vi "BuildHelpPath.vi"(1 "Help File Name":string="lvhelp.chm") -> (0 "Help File Path":path)   [LabVIEW 2018]
doc: "This VI appends the passed in file name to the help directory and returns the full path. Input defaults to LabVIEW's main help file when not supplied."
panel:
  # "This VI appends the passed in file name to the help directory and returns\nthe full path. Input defaults to LabVIEW's main help file when not supplied."
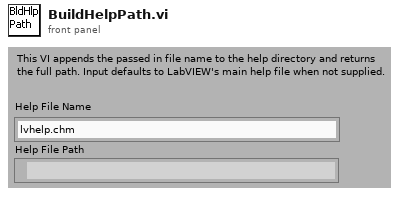
[diagram p1: front panel]
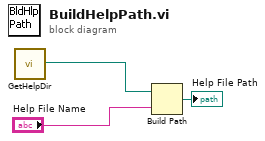
[diagram p0: block diagram]
diagram:
  n1 = call "GetHelpDir.vi"() -> ("help path"=w3:path)
  n2 = Build Path(base path=w3, name or relative path="Help File Name") -> (appended path=→"Help File Path":path)
